vi "Read CSV File.vi"(8 "error in (no error)":errorcluster, 11 "File name":string) -> (0 "error out":errorcluster, 3 "Series":u16[](array[numeric]))   [LabVIEW 2018, in "E-Series Reader.lvlib"]
doc: "Reads the specified E-Series CSV file and returns its values as a U16 array.\n\nThe VI receives the <b>File name</b> and an <b>error in</b> status. It reads the CSV file and returns the resulting values through <b>Series</b> and the resulting <b>error out</b> status."
uses:
  E-Series Reader.lvlib
  <vilib>/Utility/file.llb/Read Delimited Spreadsheet (I64).vi
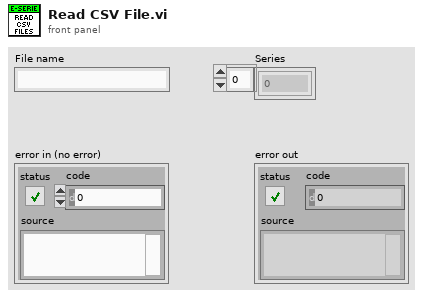
[diagram p1: front panel]
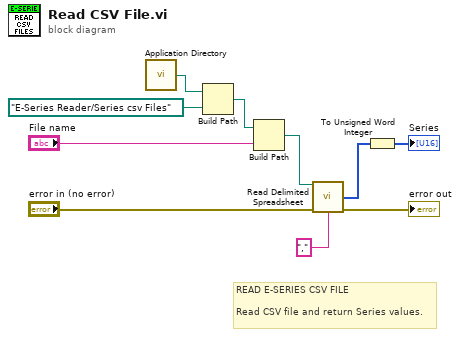
[diagram p0: block diagram]
diagram:
  # "READ E-SERIES CSV FILE\n\nRead CSV file and return Series values."
  n1 = call <vilib>:"Application Directory.vi"() -> ("Application Directory"=w3:path)
  n2 = Build Path(base path=w3, name or relative path=path "E-Series Reader/Series csv Files") -> (appended path=w1:path)
  n3 = Build Path(base path=w1, name or relative path="File name") -> (appended path=w5:path)
  n4 = call-poly <vilib>:"Read Delimited Spreadsheet.vi"("file path (dialog if empty)"=w5, "error in (no error)"="error in (no error)", "delimiter (\\t)"="," ("delimiter (\\t)")) -> ("first row"=w6:i64[], "error out"=→"error out":errorcluster)  [unwired: 7 in, 4 out]
  n5 = To Unsigned Word Integer(number=w6) -> (unsigned 16bit integer=→"Series":u16[])
